vi "Calib_General_Setup.vi"(0 "Reference instrument":T1={"high limit (10V)"=4.0, "low limit (-10V)"=0.0, "Ch No"=4, "Off ch no"=0, "Calib filename"=path "", "Ref Instrument type"=enum."Enter Value"} {"Off ch no" min=0 max=1; "Ch No" min=0 max=50; "low limit (-10V)" min=-10 max=10 format="%.1f"; "high limit (10V)" min=-10 max=10 format="%.1f"}, 1 "Requested No of samples":i32=128 min=0 step=1, 2 "Sampling rate (Hz)":sgl=1000.0 format="%.2f", 5 "2nd ref instrument":T3={"2nd Ref type"=enum."LDA", "2nd inst present"=TRUE}, 9 "Temp":dbl=20.0 format="%.1f", 12 "Abs Press (mbar)":dbl=1005.0 format="%.2f") -> (8 "Output string":string, 10 "LDA Data":bool)   [LabVIEW 2013]
uses:
  Calib_setup.ctl
  Controls/Ref_Inst_type.ctl
  Controls/Graph_Type.ctl
  Globals/Meas_global.vi
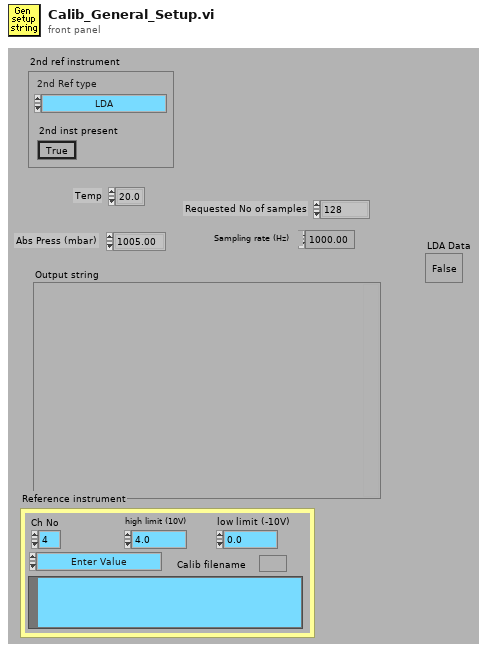
[diagram p1: front panel]
types:
  T1 = typedef "Calib_setup.ctl" = cluster{"high limit (10V)":sgl, "low limit (-10V)":sgl, "Ch No":i16, "Off ch no":i8, "Calib filename":path, "Ref Instrument type":T2}
  T2 = typedef "Ref_Inst_type.ctl" = enum16{"Propellor anemometer", "Pressure Transducer", "Raw voltage", "Pitot-static tube", "Preston tube", "Generic Linear", "Generic Polynomial", "Thermocouple", "LDA", "Enter Value", "ADAM Channel"}
  T3 = cluster{"2nd Ref type":T2, "2nd inst present":bool}
  T4 = typedef "Graph_Type.ctl" = enum16{"Show no graph", "Voltage trace", "Velocity trace", "Vel histogram", "Spectrum", "f.E(f) v Log f", "Auto-Corr"}
  T5 = cluster{"Plot 1":u16, "Plot 2":u16, "Save graph":u16, "Plot Type":T4}
  T6 = enum16{"From String to Cluster", "From Cluster to String"}
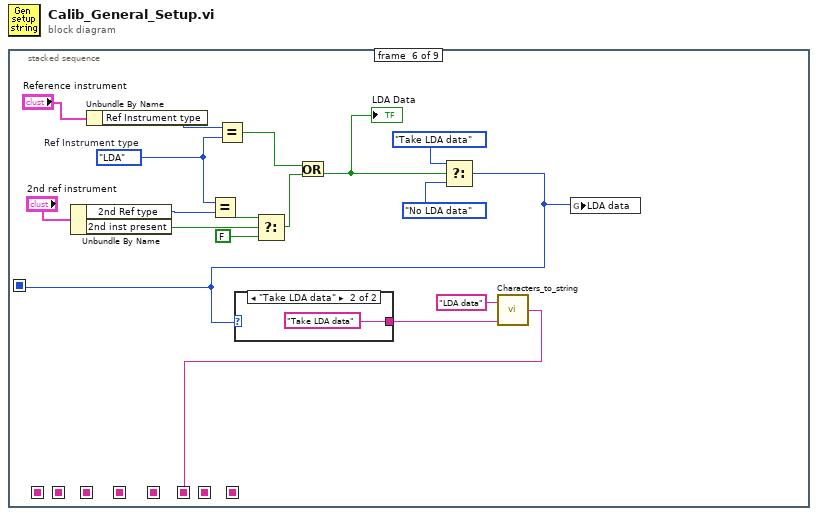
[diagram p0: block diagram]
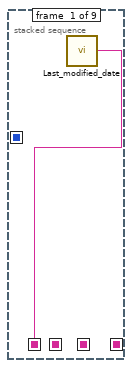
[diagram p2: hidden frame]
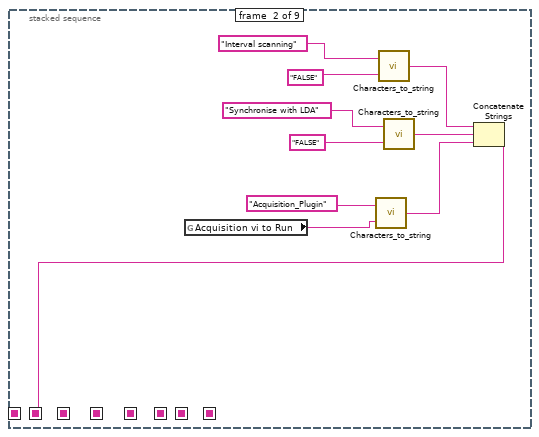
[diagram p3: hidden frame]
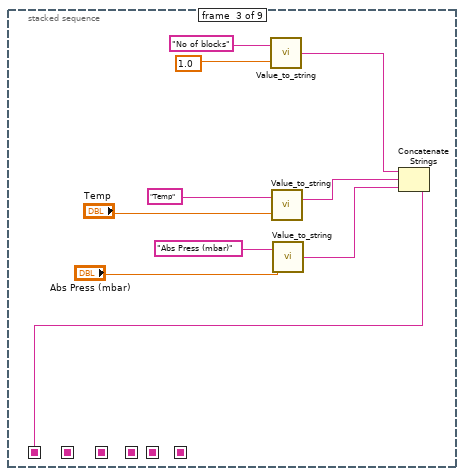
[diagram p4: hidden frame]
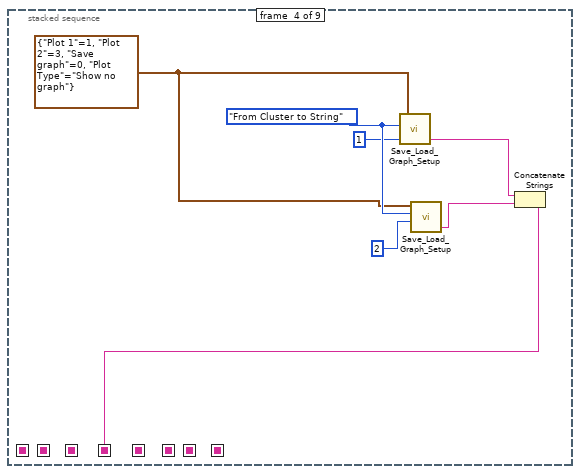
[diagram p5: hidden frame]
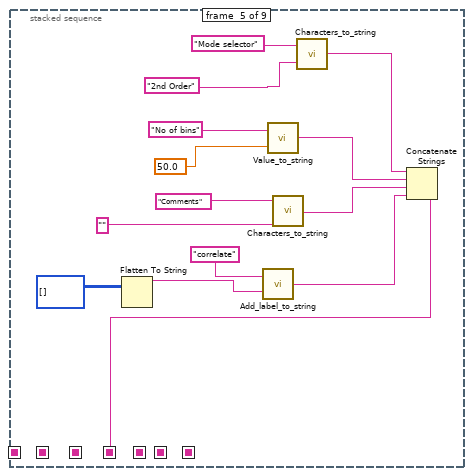
[diagram p6: hidden frame]
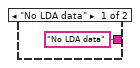
[diagram p7: hidden frame]
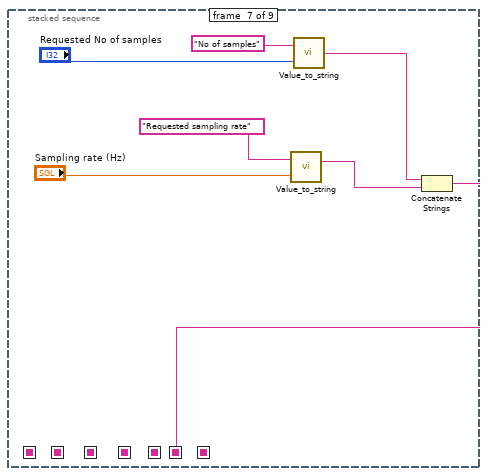
[diagram p8: hidden frame]
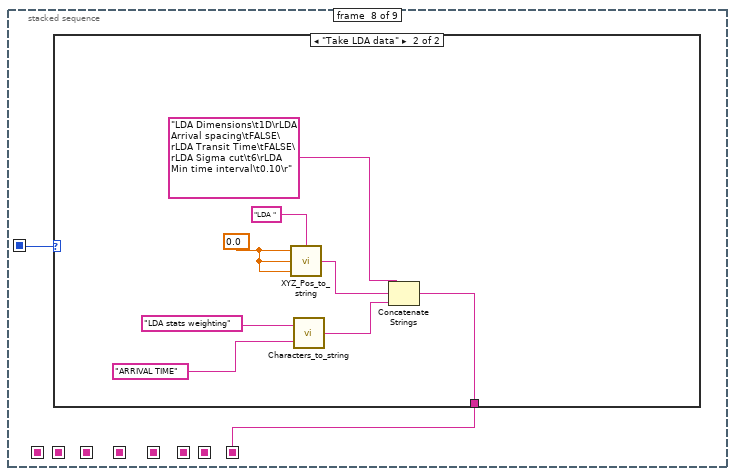
[diagram p9: hidden frame]
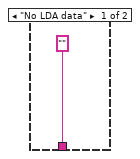
[diagram p10: hidden frame]
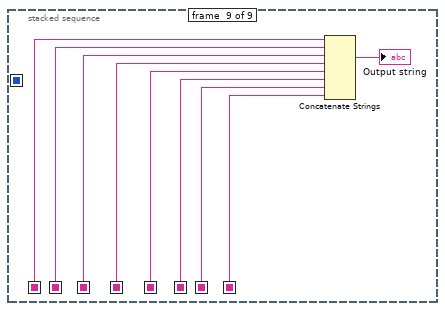
[diagram p11: hidden frame]
diagram:
  n1 = stacked-sequence {
    seq-local: [_ _ w20 _ _ _ _ _ _] -> [_ _ _ _ _ _ _ _ w88]
    seq-local: [_ w7 _ _ _ _ _ _ _] -> [_ _ _ _ _ _ _ _ w87]
    seq-local: [_ _ _ _ _ w57 _ _ _] -> [_ _ _ _ _ _ _ _ w83]
    seq-local: [_ _ _ _ _ _ w67 _ _] -> [_ _ _ _ _ _ _ _ w82]
    seq-local: [_ _ _ w23 _ _ _ _ _] -> [_ _ _ _ _ _ _ _ w85]
    seq-local: [_ _ _ _ w33 _ _ _ _] -> [_ _ _ _ _ _ _ _ w84]
    seq-local: [w1 _ _ _ _ _ _ _ _] -> [_ _ _ _ _ _ _ _ w81]
    seq-local: [_ _ _ _ _ w45 _ _ _] -> [_ _ _ _ _ _ _ w70 _]
    seq-local: [_ _ _ _ _ _ _ w69 _] -> [_ _ _ _ _ _ _ _ w80]
    frame #0 {
      n2 = call "Last_modified_date.vi"() -> ("RevisionString"=w1:string)  [unwired: 1 in, 1 out]
    }
    frame #1 {
      n3 = global read "Meas_global.vi" "Acquisition vi to Run"() -> (w3:string)
      n4 = call "Characters_to_string.vi"("Characters to write"=w3, "Label for characters"="Acquisition_Plugin") -> ("Output string"=w2:string)
      n5 = call "Characters_to_string.vi"("Characters to write"="FALSE", "Label for characters"="Interval scanning") -> ("Output string"=w9:string)
      n6 = call "Characters_to_string.vi"("Characters to write"="FALSE", "Label for characters"="Synchronise with LDA") -> ("Output string"=w8:string)
      n7 = Concatenate Strings(w9, w8, w2) -> (w7:string)
    }
    frame #2 {
      n8 = call "Value_to_string.vi"("Value"=1.0, "Label for value"="No of blocks") -> ("Output string"=w14:string)  [unwired: 1 in]
      n9 = call "Value_to_string.vi"("Value"="Temp", "Label for value"="Temp") -> ("Output string"=w17:string)  [unwired: 1 in]
      n10 = call "Value_to_string.vi"("Value"="Abs Press (mbar)", "Label for value"="Abs Press (mbar)") -> ("Output string"=w16:string)  [unwired: 1 in]
      n11 = Concatenate Strings(w14, w17, w16) -> (w20:string)
    }
    frame #3 {
      w22 = T5 {"Plot 1"=1, "Plot 2"=3, "Save graph"=0, "Plot Type"=enum."Show no graph"} ("Graph in")
      w26 = T6."From Cluster to String" ("Mode")
      n12 = call "Save_Load_Graph_Setup.vi"("Graph Number"=1, "Mode"=w26, "Graph in"=w22) -> ("Setup String Out"=w28:string)  [unwired: 1 in, 2 out]
      n13 = call "Save_Load_Graph_Setup.vi"("Graph Number"=2, "Mode"=w26, "Graph in"=w22) -> ("Setup String Out"=w27:string)  [unwired: 1 in, 2 out]
      n14 = Concatenate Strings(w28, w27) -> (w23:string)
    }
    frame #4 {
      n15 = Flatten To String(anything=i8[][] [] ("correlate")) -> (data string=w29:string)  [unwired: 1 in, 4 out]
      n16 = call "Add_label_to_string.vi"("String to write"=w29, "File Label"="correlate") -> ("Output string"=w34:string)
      n17 = call "Value_to_string.vi"("Value"=50.0 ("Bins"), "Label for value"="No of bins") -> ("Output string"=w41:string)  [unwired: 1 in]
      n18 = call "Characters_to_string.vi"("Characters to write"="" ("Comments"), "Label for characters"="Comments") -> ("Output string"=w36:string)
      n19 = call "Characters_to_string.vi"("Characters to write"="2nd Order", "Label for characters"="Mode selector") -> ("Output string"=w38:string)
      n20 = Concatenate Strings(w38, w41, w36, w34) -> (w33:string)
    }
    frame #5 {
      w44 = Ref_Inst_type."LDA"  # Ref Instrument type
      n21 = Unbundle By Name("2nd ref instrument") -> ("2nd Ref type"=w53:T2, "2nd inst present"=w54:bool)
      n22 = Unbundle By Name("Reference instrument") -> ("Ref Instrument type"=w55:T2)
      n23 = Equal?(x=w44, y=w53) -> (x = y?=w52:bool)
      n24 = Equal?(x=w55, y=w44) -> (x = y?=w49:bool)
      n25 = Select(t=w52, s=w54, f=FALSE) -> (s? t:f=w50:bool)
      n26 = Or(x=w49, y=w50) -> (x .or. y?=w46:bool)
      "LDA Data" <- w46
      n27 = Select(t=enum16{"No LDA data", "Take LDA data"}."Take LDA data" ("LDA data"), s=w46, f=enum16{"No LDA data", "Take LDA data"}."No LDA data" ("LDA data")) -> (s? t:f=w45:enum16{"No LDA data", "Take LDA data"})
      n28 = case shown="\"Take LDA data\"" w45 {
        tunnel: ["No LDA data" "Take LDA data"] -> w58
        frame "No LDA data" {
        }
        frame "Take LDA data" {
        }
      }
      n29 = call "Characters_to_string.vi"("Characters to write"=w58, "Label for characters"="LDA data") -> ("Output string"=w57:string)
      n30 = global write "Meas_global.vi" "LDA data"(w45) -> ()
    }
    frame #6 {
      n31 = call "Value_to_string.vi"("Value"="Sampling rate (Hz)", "Label for value"="Requested sampling rate") -> ("Output string"=w65:string)  [unwired: 1 in]
      n32 = call "Value_to_string.vi"("Value"="Requested No of samples", "Label for value"="No of samples") -> ("Output string"=w66:string)  [unwired: 1 in]
      n33 = Concatenate Strings(w66, w65) -> (w67:string)
    }
    frame #7 {
      n34 = case shown="\"Take LDA data\"" w70 {
        tunnel: ["" w73] -> w69
        frame "No LDA data" {
        }
        frame "Take LDA data" {
          w79 = 0.0 ("X")
          n35 = call "XYZ_Pos_to_string.vi"("Position label"="LDA ", "Z"=w79, "Y"=w79, "X"=w79) -> ("Output string"=w75:string)
          n36 = call "Characters_to_string.vi"("Characters to write"="ARRIVAL TIME" ("LDA stats type"), "Label for characters"="LDA stats weighting") -> ("Output string"=w74:string)
          n37 = Concatenate Strings("LDA Dimensions\t1D\rLDA Arrival spacing\tFALSE\rLDA Transit Time\tFALSE\rLDA Sigma cut\t6\rLDA Min time interval\t0.10\r" ("String"), w75, w74) -> (w73:string)
        }
      }
    }
    frame #8 {
      n38 = Concatenate Strings(w81, w87, w88, w85, w84, w83, w82, w80) -> (→"Output string":string)
    }
  }
